vi "serial read.vi"() -> ()   [LabVIEW 2017]
uses:
  <vilib>/Instr/_visa.llb/VISA Configure Serial Port (Instr).vi
panel:
  in  "Slide 2":dbl(slide) scale=0.0..1000.0
  in  "write buffer":string
  in  "baud rate (9600)":u32=9600
  out "read buffer":string
  out "Loop Number":i32
  in  "stop":bool
  in  "COM":refnum<visa-resource-name>
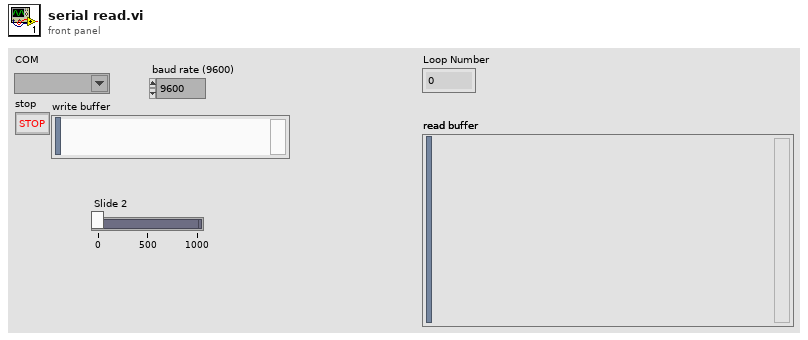
[diagram p1: front panel]
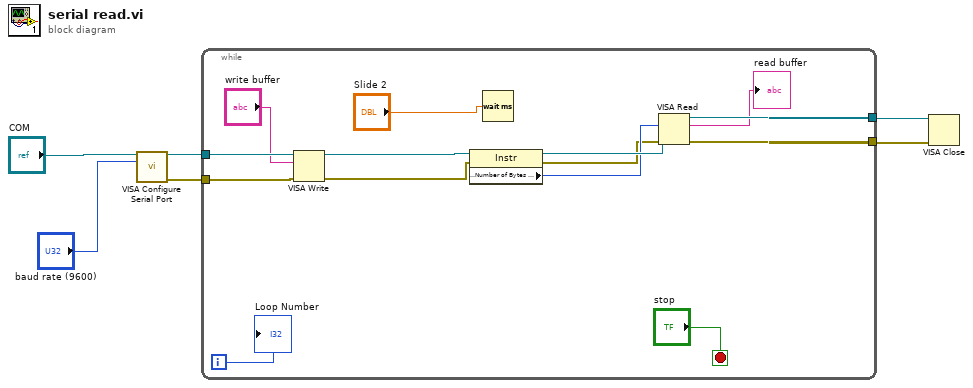
[diagram p0: block diagram]
diagram:
  n1 = call-poly "VISA Configure Serial Port"("VISA resource name"="COM", "baud rate (9600)"="baud rate (9600)") -> ("VISA resource name out"=w5:refnum<visa-resource-name>, "error out"=w6:errorcluster)  [unwired: 12 in]
  n2 = while {
    tunnel: w6 -> [w17]
    tunnel: w5 -> [w18]
    tunnel: [w12] -> w2
    tunnel: [w11] -> w1
    i -> [w19]
    stop <- "stop" stop-if-true
    n3 = VISA Write(VISA resource name=w18, write buffer="write buffer", error in (no error)=w17) -> (VISA resource name out=w16:refnum<visa-resource-name>, error out=w15:errorcluster)  [unwired: 1 out]
    n4 = property class="Instr"(reference=w16, error in=w15) -> (reference out=w14:refnum<visa-resource-name>, error out=w8:errorcluster, "Serial Settings:Number of Bytes at Serial Port"=w13:u32)
    n5 = Wait (ms)(milliseconds to wait="Slide 2") -> ()  [unwired: 1 out]
    n6 = VISA Read(VISA resource name=w14, byte count=w13, error in (no error)=w8) -> (VISA resource name out=w12:refnum<visa-resource-name>, read buffer=→"read buffer":string, error out=w11:errorcluster)  [unwired: 1 out]
    "Loop Number" <- w19
  }
  n7 = VISA Close(VISA resource name=w2, error in (no error)=w1) -> ()  [unwired: 1 out]
